vi "Overlay Delete Elements in Properties Tree.vi"(8 "error in":errorcluster, 10 "Prior Property Array":T1(array[cluster]), 11 "Tree Ref":refnum<vi>) -> (0 "error out":errorcluster, 3 "Tree Ref Out":refnum<vi>)   [LabVIEW 2023]
panel:
  out "exe time (ms)":u32
  in  "Tree":string[](tree)
  # "1ms per affected row"
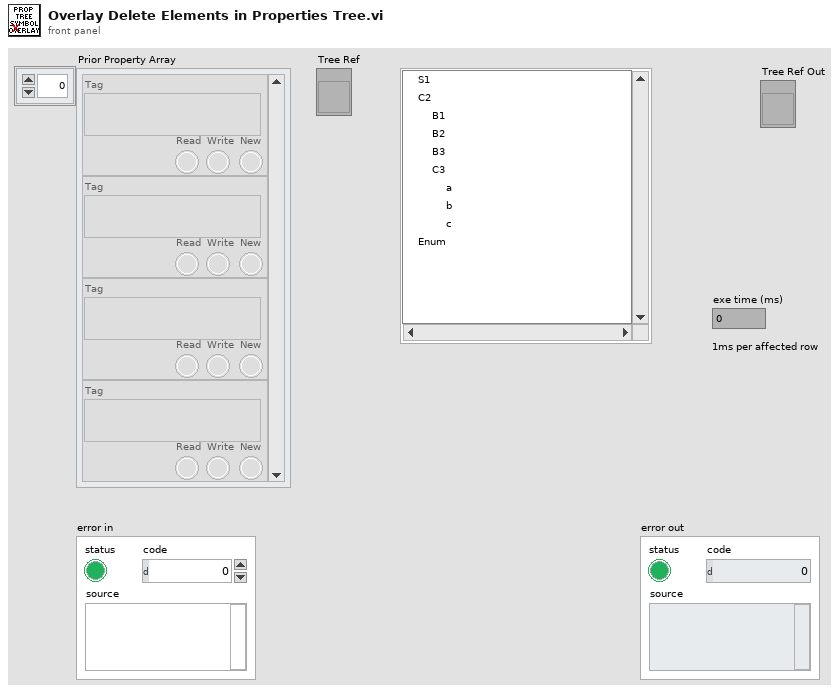
[diagram p1: front panel]
types:
  T1 = cluster{"Tag":string, "Read":bool, "Write":bool, "New":bool}[]
  T2 = enum16{"Init", "Read", "Remove", "Remove or Append", "Append", "Append If New"}
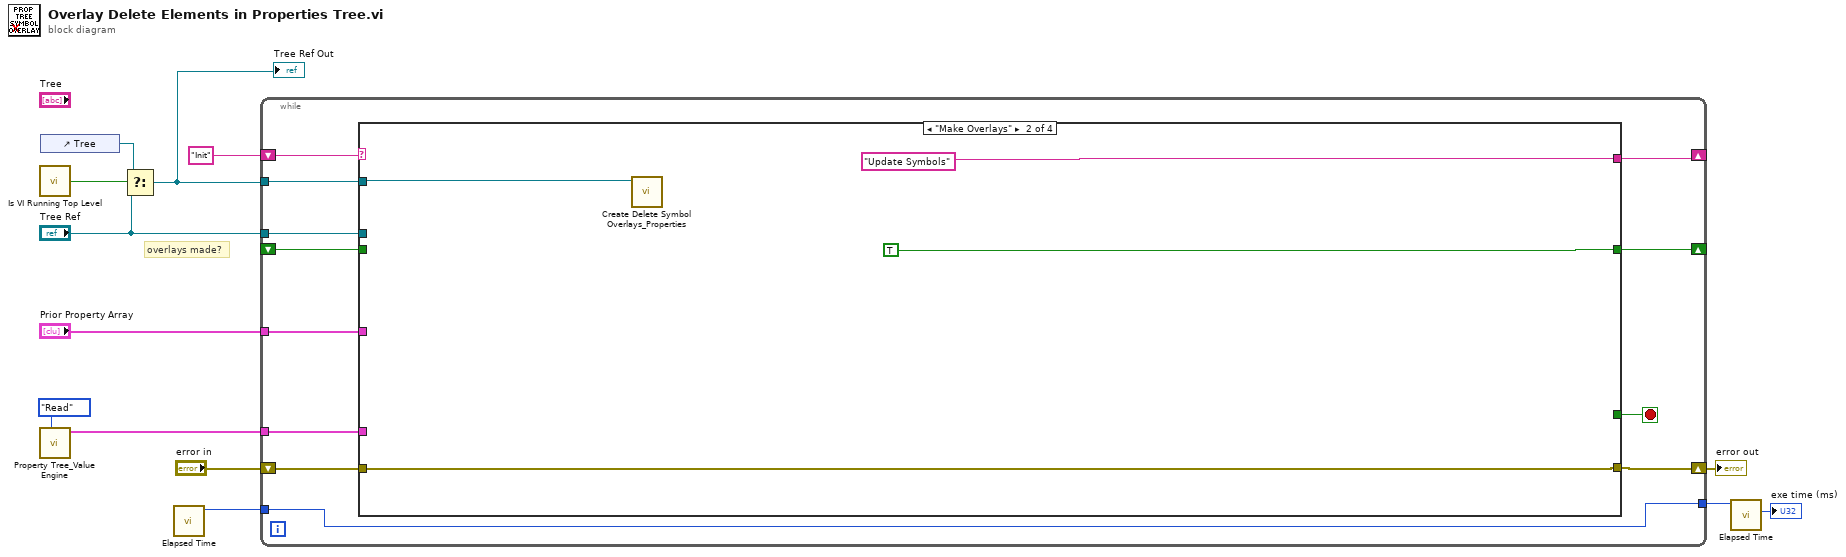
[diagram p0: block diagram]
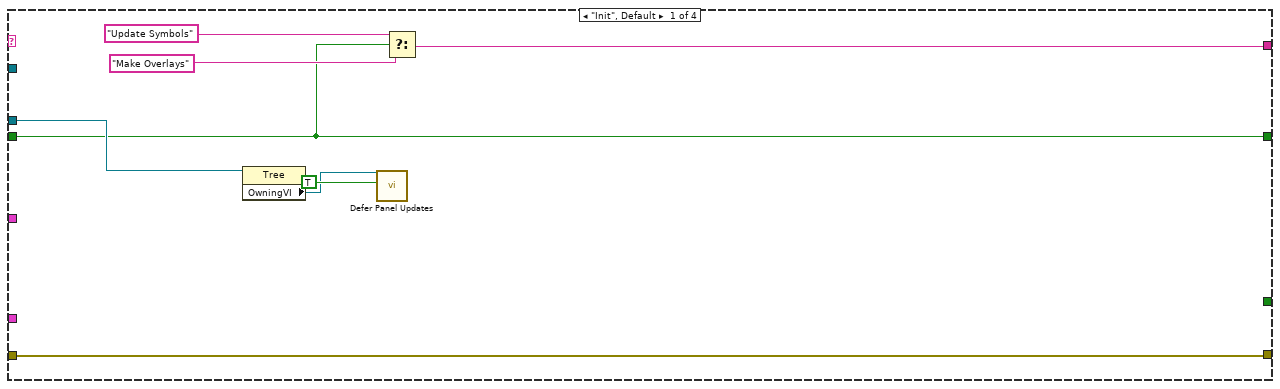
[diagram p2: hidden frame]
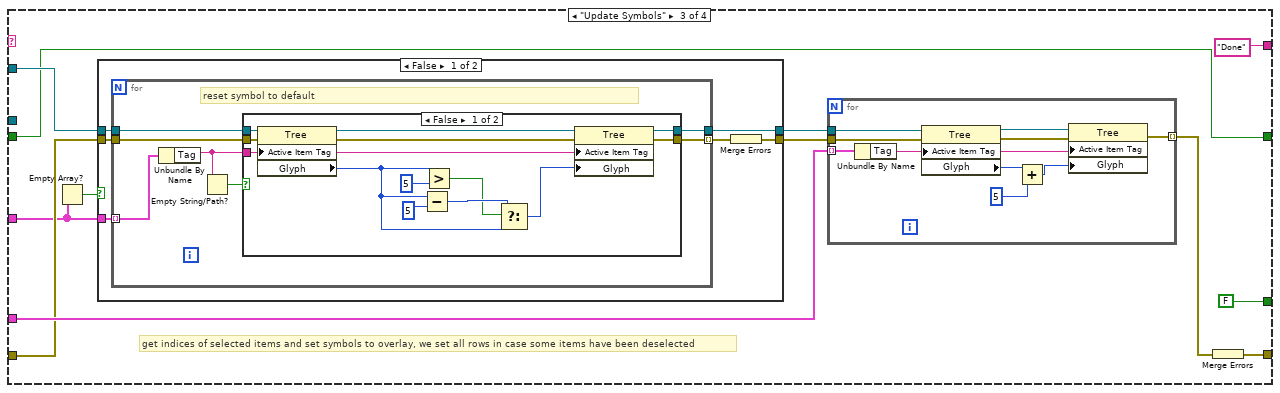
[diagram p3: hidden frame]
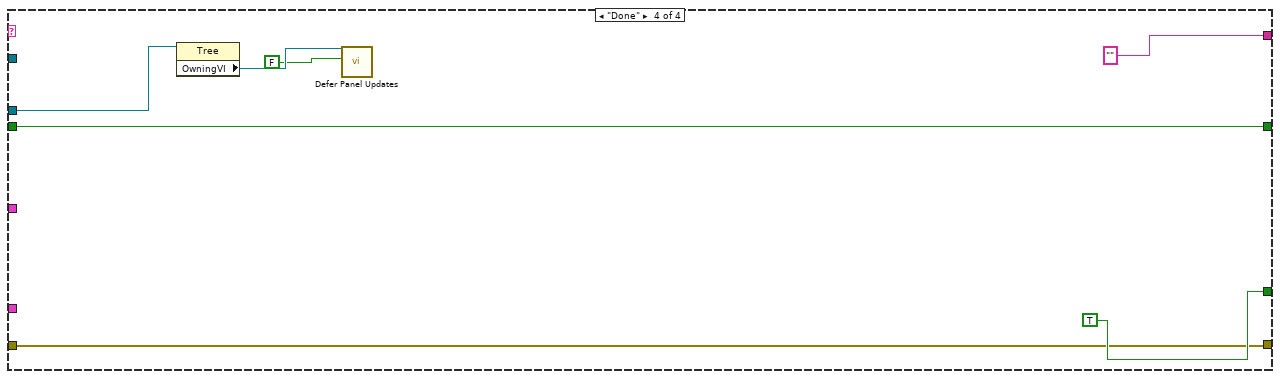
[diagram p6: hidden frame]
diagram:
  # "overlays made?"
  n1 = call "Is VI Running Top Level.vi"() -> ("Top Level?"=w13:bool)  [unwired: 5 in]
  n2 = call "Property Tree_Value Engine.vi"("Save Action"=T2."Read" ("Action")) -> ("Property Array Out"=w4:T1)  [unwired: 8 in, 2 out]
  n3 = control-ref of="Tree"() -> (w12:refnum<vi>)
  n4 = Select(t=w12, s=w13, f="Tree Ref") -> (s? t:f=w10:refnum<vi>)
  "Tree Ref Out" <- w10
  n5 = call "Elapsed Time.vi"() -> ("millisecond timer value"=w8:u32)  [unwired: 7 in, 4 out]
  n6 = while {
    tunnel: w10 -> [w25]
    shift-right: [w23] -> _
    shift-left: "Init" -> [w24]
    shift-right: [w22] -> _
    shift-left: _ -> [w21]
    tunnel: [w19] -> w9
    tunnel: w8 -> [w19]
    tunnel: "Prior Property Array" -> [w18]
    tunnel: w4 -> [w17]
    tunnel: "Tree Ref" -> [w16]
    shift-right: [w14] -> w1
    shift-left: "error in" -> [w15]
    stop <- w20 stop-if-true
    n7 = case shown="\"Make Overlays\"" w24 {
      tunnel: w25 -> [_ w35 w49 _]
      tunnel: w21 -> [w27 _ w48 w90]
      tunnel: [w33 "Update Symbols" "Done" ""] -> w23
      tunnel: [w27 TRUE w48 w90] -> w22
      tunnel: [_ _ FALSE TRUE] -> w20
      tunnel: w18 -> [_ _ w39 _]
      tunnel: w17 -> [_ _ w45 _]
      tunnel: w16 -> [w29 _ _ w93]
      tunnel: w15 -> [w26 w34 w43 w89]
      tunnel: [w26 w34 w40 w89] -> w14
      frame "Init", Default {
        n8 = property class="Tree"(reference=w29) -> ("OwningVI"=w28:refnum<vi>)  [unwired: 1 in, 2 out]
        n9 = call "Defer Panel Updates.vi"("Defer Panel Updates [T]"=TRUE, "VI Ref"=w28) -> ()  [unwired: 8 in, 2 out]
        n10 = Select(t="Update Symbols", s=w27, f="Make Overlays") -> (s? t:f=w33:string)
      }
      frame "Make Overlays" {
        n11 = call "Create Delete Symbol Overlays_Properties.vi"("Tree Ref"=w35) -> ()  [unwired: 11 in]
      }
      frame "Update Symbols" {
        # "get indices of selected items and set symbols to overlay, we set all rows in case some items have been deselected"
        n12 = Empty Array?(array=w39) -> (empty?=w38:bool)
        n13 = case shown="False" w38 {
          tunnel: w49 -> [w55 w78]
          tunnel: [w54 w78] -> w46
          tunnel: w39 -> [w53 _]
          tunnel: w43 -> [w52 w77]
          tunnel: [w50 w77] -> w41
          frame False {
            n14 = for {
              tunnel: w55 -> [w62]
              tunnel: [w61] -> w54
              tunnel: w53 -> [w60] mode=indexing
              tunnel: w52 -> [w59]
              tunnel: [w58] -> w51 mode=indexing
              # "reset symbol to default"
              n15 = Unbundle By Name(w60) -> ("Tag"=w57:string)
              n16 = Empty String/Path?(string/path=w57) -> (empty?=w56:bool)
              n17 = case shown="False" w56 {
                tunnel: w62 -> [w74 w76]
                tunnel: [w68 w76] -> w61
                tunnel: w57 -> [w67 _]
                tunnel: w59 -> [w66 w75]
                tunnel: [w64 w75] -> w58
                frame False {
                  n18 = property class="Tree"(reference=w74, error in=w66, "Active Item Tag"=w67) -> (error out=w65:errorcluster, "Glyph"=w69:i32)  [unwired: 1 out]
                  n19 = Subtract(x=w69, y=5) -> (x-y=w72:i32)
                  n20 = Greater?(x=w69, y=5) -> (0:w71:bool)
                  n21 = Select(t=w72, s=w71, f=w69) -> (s? t:f=w70:i32)
                  n22 = property class="Tree"(reference=w74, error in=w65, "Active Item Tag"=w67, "Glyph"=w70) -> (reference out=w68:refnum<vi>, error out=w64:errorcluster)
                }
                frame True {
                  # "#revisit not sure why we get blank items in value array"
                }
              }
            }
            n23 = Merge Errors(w51) -> (w50:errorcluster)
          }
          frame True {
          }
        }
        n24 = for {
          tunnel: w46 -> [w88]
          tunnel: w45 -> [w83] mode=indexing
          tunnel: w41 -> [w81]
          tunnel: [w79] -> w42 mode=indexing
          n25 = Unbundle By Name(w83) -> ("Tag"=w82:string)
          n26 = property class="Tree"(reference=w88, error in=w81, "Active Item Tag"=w82) -> (reference out=w87:refnum<vi>, error out=w80:errorcluster, "Glyph"=w86:i32)
          n27 = Add(x=w86, y=5) -> (x+y=w85:i32)
          n28 = property class="Tree"(reference=w87, error in=w80, "Active Item Tag"=w82, "Glyph"=w85) -> (error out=w79:errorcluster)  [unwired: 1 out]
        }
        n29 = Merge Errors(w42) -> (w40:errorcluster)
      }
      frame "Done" {
        n30 = property class="Tree"(reference=w93) -> ("OwningVI"=w95:refnum<vi>)  [unwired: 1 in, 2 out]
        n31 = call "Defer Panel Updates.vi"("Defer Panel Updates [T]"=FALSE, "VI Ref"=w95) -> ()  [unwired: 8 in, 2 out]
      }
    }
  }
  "error out" <- w1
  n32 = call "Elapsed Time.vi"("past time"=w9) -> ("elapsed time (ms)"=→"exe time (ms)":u32)  [unwired: 6 in, 4 out]
